vi "ConnectTerminals.vi"() -> ()   [LabVIEW 2018]
panel:
  in  "Ring":u16(ring)=1 items=["Connect", "Disconnect"]
  in  "output terminal":tag="/6733_1/PXI_Trig0"
  in  "source terminal":tag="/6733_1/PFI0"
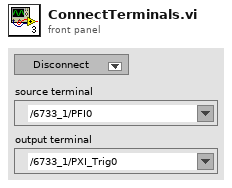
[diagram p1: front panel]
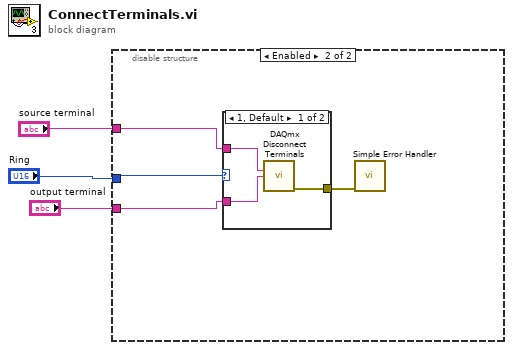
[diagram p0: block diagram]
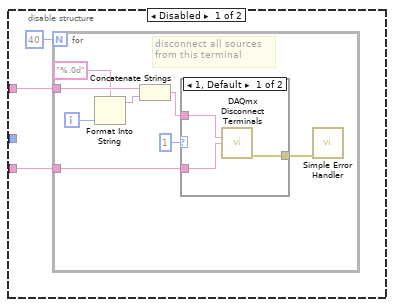
[diagram p2: hidden frame]
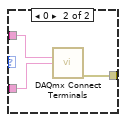
[diagram p3: hidden frame]
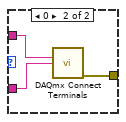
[diagram p4: hidden frame]
diagram:
  n1 = disable-structure shown="Enabled" {
    disable-tunnel: "output terminal" -> [w6 w22]
    disable-tunnel: "Ring" -> [_ w21]
    disable-tunnel: "source terminal" -> [w5 w23]
    frame Disabled {
      n2 = for {
        N: 40 -> [_]
        tunnel: w6 -> [w14]
        tunnel: w5 -> [w12]
        i -> [w10]
        # "disconnect all sources \nfrom this terminal"
        n3 = Format Into String(format string="%.0d", w10) -> (resulting string=w11:string)  [unwired: 2 in, 1 out]
        n4 = Concatenate Strings(w12, w11) -> (w8:string)
        n5 = case shown="1, Default" u16 1 ("Ring") {
          tunnel: w8 -> [w17 w20]
          tunnel: w14 -> [w16 w19]
          tunnel: [w15 w18] -> w13
          frame 1, Default {
            n6 = call <vilib>:"DAQmx Disconnect Terminals.vi"("source terminal"=w17, "destination terminal"=w16) -> ("error out"=w15:errorcluster)  [unwired: 13 in]
          }
          frame 0 {
            n7 = call <vilib>:"DAQmx Connect Terminals.vi"("source terminal"=w20, "destination terminal"=w19) -> ("error out"=w18:errorcluster)  [unwired: 13 in]
          }
        }
        n8 = call <vilib>:"Simple Error Handler.vi"("error in (no error)"=w13) -> ()  [unwired: 4 in, 5 out]
      }
    }
    frame Enabled {
      n9 = case shown="1, Default" w21 {
        tunnel: w23 -> [w27 w30]
        tunnel: w22 -> [w26 w29]
        tunnel: [w25 w28] -> w24
        frame 1, Default {
          n10 = call <vilib>:"DAQmx Disconnect Terminals.vi"("source terminal"=w27, "destination terminal"=w26) -> ("error out"=w25:errorcluster)  [unwired: 13 in]
        }
        frame 0 {
          n11 = call <vilib>:"DAQmx Connect Terminals.vi"("source terminal"=w30, "destination terminal"=w29) -> ("error out"=w28:errorcluster)  [unwired: 13 in]
        }
      }
      n12 = call <vilib>:"Simple Error Handler.vi"("error in (no error)"=w24) -> ()  [unwired: 4 in, 5 out]
    }
  }
